vi "Task interface-Trial start DO flag.vi"(7 "Function":T1, 8 "error in":errorcluster, 10 "DO value":bool) -> (0 "error out":errorcluster)   [LabVIEW 2013]
uses:
  typedefs/Functions enum.ctl
  Typedefs/HW config states enum.ctl
  <vilib>/DAQmx/write.llb/DAQmx Write.vi
  <vilib>/DAQmx/write.llb/DAQmx Write (Digital Bool 1Line 1Point).vi
  <vilib>/DAQmx/create/channels.llb/DAQmx Create Channel (DO-Digital Output).vi
  <vilib>/DAQmx/miscellaneous.llb/DAQmx Fill In Error Info.vi
panel:
  out "\"Start trial\" flag DO channel":tag="PXI1Slot4/port0/line7"
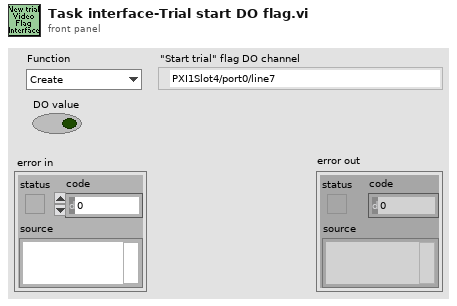
[diagram p1: front panel]
types:
  T1 = typedef "Functions enum.ctl" = enum16{"Create", "Start", "Write", "Stop", "Clear"}
  T2 = typedef "HW config states enum.ctl" = enum16{"Load from file", "Save to file", "Write all", "Read all", "Write XY stage settings", "Write DAQ FPGA settings", "Write Control FPGA settings", "Write Phys Channels", "Clear", "Compare from file"}
  T3 = typedef "Sys Configuration.ctl" = cluster{"XY Stage":T4, "DAQ FPGA":T5, "Control system":T9, "Encoder":T10, "DAQmx Chan":T11, "Computer MAC address":string, "Cam VidRec":T12, "Externalise Triggers":bool, "Laser wavelength (nm)":dbl}
  T4 = typedef "XY Stage config cluster.ctl" = cluster{"COM port":refnum<visa-resource-name>, "XY stage available":bool}
  T5 = typedef "DAQ FPGA config cluster.ctl" = cluster{"Ref":T6, "Target":T7, "Clock Freq (MHz) ":dbl, "input card type":T8, "Samples Wait after Trigger":u16, "AOD fill":u16, "StartupDelay":i32, "Slip Cycle (clock cycles)":u32, "Add Cycle":bool}
  T6 = typedef "FPGA Ref.ctl" = refnum<k20>
  T7 = typedef "nirio_resource_hc.ctl" = tag
  T8 = typedef "FPGA input type AC-DC.ctl" = enum16{"AC Card", "DC Card"}
  T9 = typedef "CTRL system config cluster.ctl" = cluster{"Ethernet opened":bool, "Ethernet Port":u32, "Ctrl FPGA available":bool, "Ctrl FPGA Clock (MHz)":dbl, "Ctrl system MAC address":string, "Control system.Network adapter name":string, "AOD 1 Amplitude":i16, "AOD 2 Amplitude":i16, "AOD 3 Amplitude":i16, "AOD 4 Amplitude":i16, "Data Time Interval (ns)":dbl, "T0 (ns)":dbl, "Ta (ns)":dbl}
  T10 = typedef "Encoder config cluster.ctl" = cluster{"IP address":string, "Port":u16, "Encoder available":bool, "Wheel radius (cm)":dbl}
  T11 = typedef "DAQmx physical channels cluster.ctl" = cluster{"Pockels AO":tag, "Hard shutter AO":tag, "PMT AOs":tag, "Power meter AI":tag}
  T12 = typedef "Cam VidRec HW config setup cluster.ctl" = cluster{"DO flag-Video record":tag, "DO flag-Trial start":tag, "VidRec available":bool}
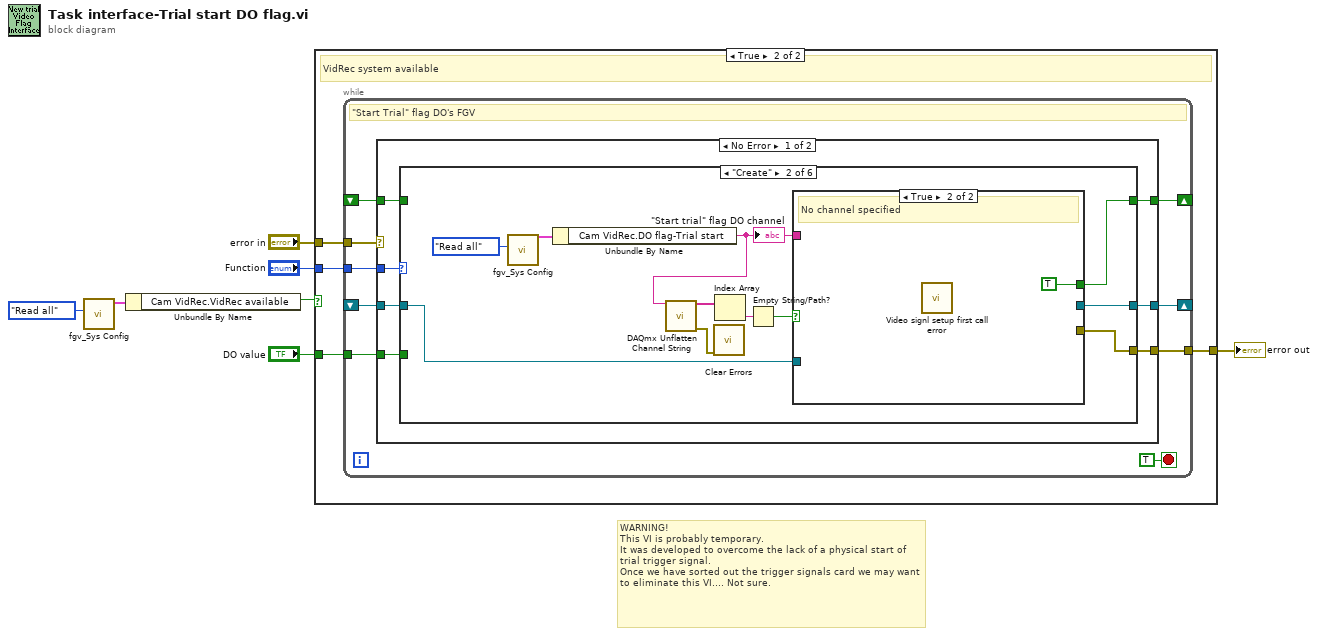
[diagram p0: block diagram]
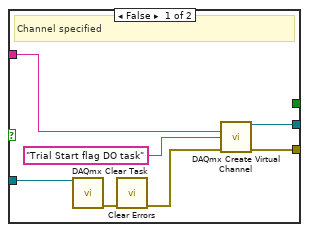
[diagram p4: hidden frame]
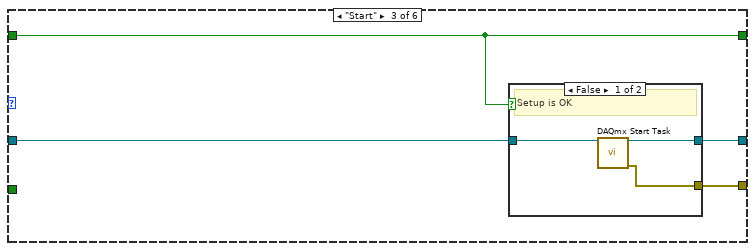
[diagram p5: hidden frame]
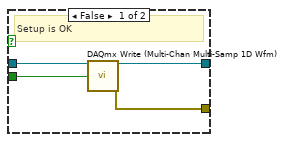
[diagram p8: hidden frame]
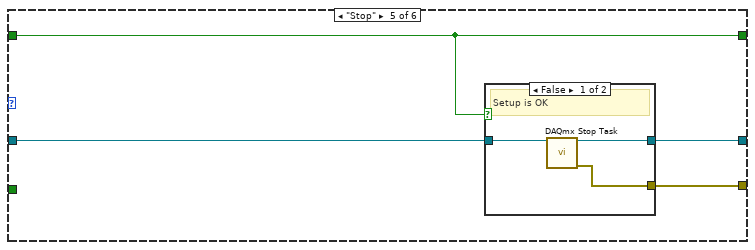
[diagram p9: hidden frame]
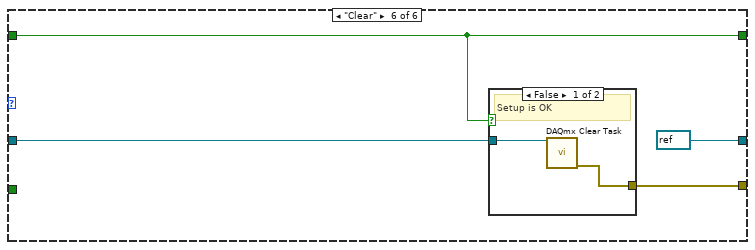
[diagram p11: hidden frame]
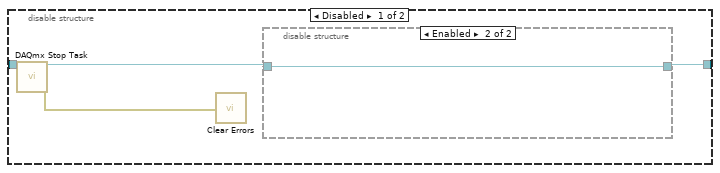
[diagram p14: hidden frame]
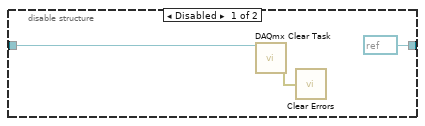
[diagram p15: hidden frame]
diagram:
  # "WARNING!\nThis VI is probably temporary.\nIt was developed to overcome the lack of a physical start of trial trigger signal.\nOnce we have sorted out the trigger signals card we may want to eliminate this VI.... Not sure."
  n1 = call "fgv_Sys Config.vi"("Function"=HW_config_states_enum."Read all") -> ("System Config out"=w2:T3)  [unwired: 9 in, 1 out]
  n2 = Unbundle By Name(w2) -> ("Cam VidRec.VidRec available"=w1:bool)
  n3 = case shown="True" w1 {
    tunnel: "Function" -> [_ w12]
    tunnel: "DO value" -> [_ w11]
    tunnel: [w8 w10] -> w5
    tunnel: "error in" -> [w8 w9]
    frame False {
      # "VidRec system unavailable"
    }
    frame True {
      # "VidRec system available"
      n4 = while {
        tunnel: [w20] -> w10
        shift-right: [w21] -> _
        shift-left: _ -> [w19]
        tunnel: w12 -> [w18]
        tunnel: w11 -> [w17]
        tunnel: w9 -> [w15]
        shift-right: [w14] -> _
        shift-left: _ -> [w13]
        stop <- TRUE stop-if-true
        # "\"Start Trial\" flag DO's FGV"
        n5 = case shown="No Error" w15 {
          selector: w15 -> [_ w84]
          tunnel: [w28 w83] -> w21
          tunnel: [w27 w84] -> w20
          tunnel: w19 -> [w26 w85]
          tunnel: w18 -> [w25 _]
          tunnel: w17 -> [w24 _]
          tunnel: [w23 w82] -> w14
          tunnel: w13 -> [w22 w82]
          frame No Error {
            n6 = case shown="\"Create\"" w25 {
              tunnel: [w30 w41 w52 w61 w70 refnum<k21> refnum ("task out")] -> w28
              tunnel: [_ w40 w51 w60 w69 w77] -> w27
              tunnel: w26 -> [w30 w38 w53 w62 w71 w79]
              tunnel: w24 -> [_ _ _ w59 _ _]
              tunnel: [w29 w34 w50 w58 w68 w76] -> w23
              tunnel: w22 -> [w29 _ w50 w58 w68 w76]
              frame Default {
              }
              frame "Create" {
                n7 = call "fgv_Sys Config.vi"("Function"=HW_config_states_enum."Read all") -> ("System Config out"=w33:T3)  [unwired: 9 in, 1 out]
                n8 = Unbundle By Name(w33) -> ("Cam VidRec.DO flag-Trial start"=w31:tag)
                "\"Start trial\" flag DO channel" <- w31
                n9 = call <vilib>:"DAQmx Unflatten Channel String.vi"("names in"=w31) -> ("names out"=w39:string[], "error out"=w35:errorcluster)  [unwired: 13 in]
                n10 = call <vilib>:"Clear Errors.vi"("error in (no error)"=w35) -> ()  [unwired: 6 in, 1 out]
                n11 = Index Array(array=w39) -> (element=w37:string)  [unwired: 1 in]
                n12 = Empty String/Path?(string/path=w37) -> (empty?=w36:bool)
                n13 = case shown="True" w36 {
                  tunnel: [w48 _] -> w41
                  tunnel: [w44 _] -> w40
                  tunnel: w38 -> [w43 _]
                  tunnel: [_ TRUE ("Disabled")] -> w34
                  tunnel: w31 -> [w42 _]
                  frame False {
                    # "Channel specified"
                    n14 = call <vilib>:"DAQmx Clear Task.vi"("task in"=w43) -> ("error out"=w46:errorcluster)  [unwired: 14 in]
                    n15 = call <vilib>:"Clear Errors.vi"("error in (no error)"=w46) -> ("error out"=w45:errorcluster)  [unwired: 6 in]
                    n16 = call-poly <vilib>:"DAQmx Create Virtual Channel.vi"("lines"=w42, "name to assign"="Trial Start flag DO task", "error in"=w45) -> ("task out"=w48:refnum<k21>, "error out"=w44:errorcluster)  [unwired: 11 in]
                  }
                  frame True {
                    # "No channel specified"
                    n17 = call "Video signl setup first call error.vi"() -> ()  [unwired: 12 in]
                  }
                }
              }
              frame "Start" {
                n18 = case shown="False" w50 {
                  tunnel: w53 -> [w56 w57]
                  tunnel: [w55 w57] -> w52
                  tunnel: [w54 _] -> w51
                  frame False {
                    # "Setup is OK"
                    n19 = call <vilib>:"DAQmx Start Task.vi"("task/channels in"=w56) -> ("task out"=w55:refnum<k21>, "error out"=w54:errorcluster)  [unwired: 13 in]
                  }
                  frame True {
                    # "Disabled due to bad setup"
                  }
                }
              }
              frame "Write" {
                n20 = case shown="True" w58 {
                  tunnel: w62 -> [w66 w67]
                  tunnel: [w65 w67] -> w61
                  tunnel: [w64 _] -> w60
                  tunnel: w59 -> [w63 _]
                  frame False {
                    # "Setup is OK"
                    n21 = call-poly "DAQmx Write (Multi-Chan Multi-Samp 1D Wfm).vi"("task/channels in"=w66, "data"=w63) -> ("task out"=w65:refnum<k21>, "error out"=w64:errorcluster)  [unwired: 11 in, 1 out]
                  }
                  frame True {
                    # "Disabled due to bad setup"
                  }
                }
              }
              frame "Stop" {
                n22 = case shown="False" w68 {
                  tunnel: w71 -> [w74 w75]
                  tunnel: [w73 w75] -> w70
                  tunnel: [w72 _] -> w69
                  frame False {
                    # "Setup is OK"
                    n23 = call <vilib>:"DAQmx Stop Task.vi"("task/channels in"=w74) -> ("task out"=w73:refnum<k21>, "error out"=w72:errorcluster)  [unwired: 13 in]
                  }
                  frame True {
                    # "Disabled due to bad setup"
                  }
                }
              }
              frame "Clear" {
                n24 = case shown="False" w76 {
                  tunnel: w79 -> [w81 _]
                  tunnel: [w80 _] -> w77
                  frame False {
                    # "Setup is OK"
                    n25 = call <vilib>:"DAQmx Clear Task.vi"("task in"=w81) -> ("error out"=w80:errorcluster)  [unwired: 14 in]
                  }
                  frame True {
                    # "Disabled due to bad setup"
                  }
                }
              }
            }
          }
          frame Error {
            n26 = disable-structure shown="Enabled" {
              disable-tunnel: w85 -> [w88 w94]
              disable-tunnel: [w86 w94] -> w83
              frame Disabled {
                n27 = call <vilib>:"DAQmx Stop Task.vi"("task/channels in"=w88) -> ("task out"=w89:refnum<k21>, "error out"=w87:errorcluster)  [unwired: 13 in]
                n28 = call <vilib>:"Clear Errors.vi"("error in (no error)"=w87) -> ()  [unwired: 6 in, 1 out]
                n29 = disable-structure shown="Enabled" {
                  disable-tunnel: w89 -> [w92 w93]
                  disable-tunnel: [refnum<k21> refnum ("task out") w93] -> w86
                  frame Disabled {
                    n30 = call <vilib>:"DAQmx Clear Task.vi"("task in"=w92) -> ("error out"=w91:errorcluster)  [unwired: 14 in]
                    n31 = call <vilib>:"Clear Errors.vi"("error in (no error)"=w91) -> ()  [unwired: 6 in, 1 out]
                  }
                  frame Enabled {
                  }
                }
              }
              frame Enabled {
              }
            }
          }
        }
      }
    }
  }
  "error out" <- w5
